vi "Atto DRY Interface set Derivative Gain.vi"(8 "error in (no error)":errorcluster, 11 "DerivativeGain":sgl) -> (0 "error out":errorcluster, 3 "function return":i32)   [LabVIEW 2016, in "attoDRYLib.lvlib"]
doc: "int32_t __cdecl AttoDRY_Interface_setDerivativeGain(float DerivativeGain);"
uses:
  <userlib>/attoDRYLib/attoDRYLib.lvlib
  <userlib>/attoDRYLib/attoDRYLib.dll
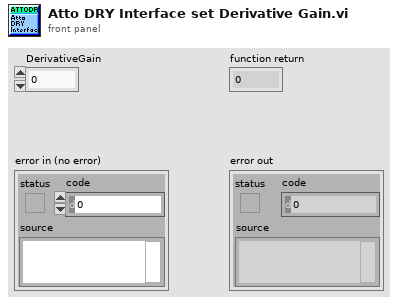
[diagram p1: front panel]
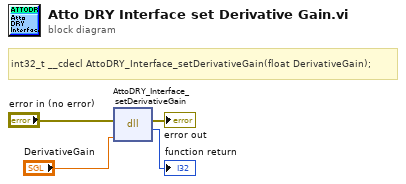
[diagram p0: block diagram]
diagram:
  # "int32_t __cdecl AttoDRY_Interface_setDerivativeGain(float DerivativeGain);"
  n1 = dll-call lib="C:/Program Files (x86)/National Instruments/LabVIEW 2016/user.lib/attoDRYLib/attoDRYLib.*" fn="AttoDRY_Interface_setDerivativeGain"(error in="error in (no error)", "DerivativeGain"="DerivativeGain") -> (error out=→"error out":errorcluster, →"function return":i32)  [unwired: 3 in, 1 out]
